vi "max and min of domain and freq.vi"() -> ()   [LabVIEW 2017]
uses:
  <vilib>/measure/maspectr.llb/FFT Power Spectrum and PSD for 1 Chan.vi
  <vilib>/measure/NI_MAPro.lvlib
panel:
  out "min value freq":dbl
  out "max value freq":dbl
  out "main signal":waveform(dbl)[](graph)
  out "power spectrum":cluster{"f0":dbl, "df":dbl, "magnitude":dbl[]}(graph)
  out "min value domain":dbl
  out "max value domain":dbl
  in  "path 4":path
  in  "path 3":path
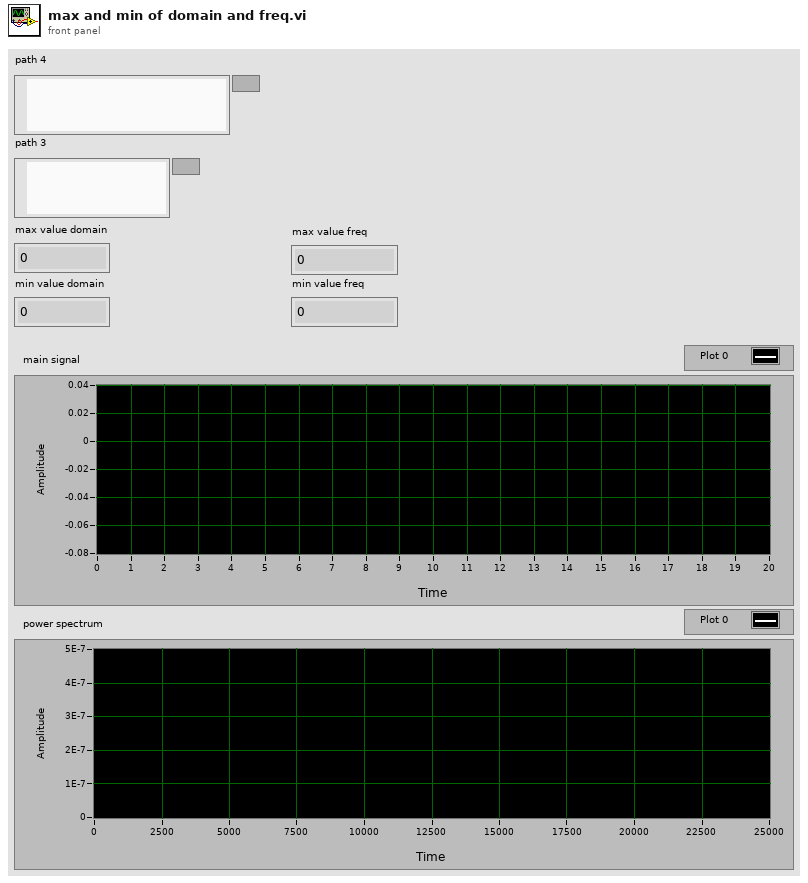
[diagram p1: front panel]
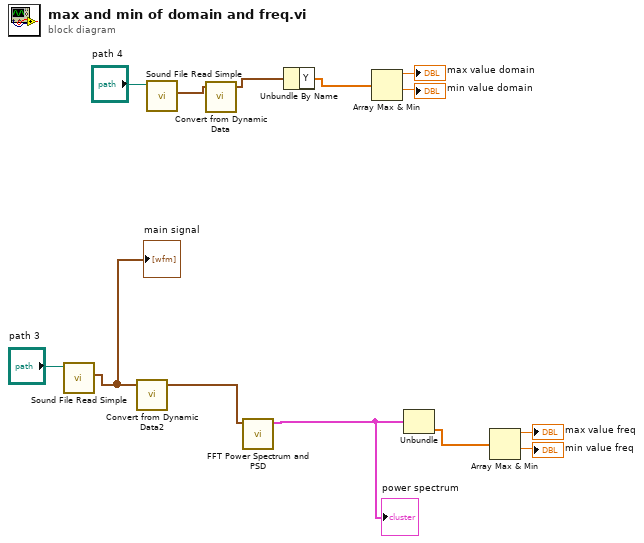
[diagram p0: block diagram]
diagram:
  n1 = call <vilib>:"Sound File Read Simple.vi"("path"="path 3") -> ("data"=w4:waveform(dbl)[])  [unwired: 7 in, 3 out]
  "main signal" <- w4
  n2 = call "Convert from Dynamic Data2"("Dynamic Data Type"=w4) -> ("Waveform"=w6:waveform(dbl))  [unwired: 3 in]
  n3 = call <vilib>:"Sound File Read Simple.vi"("path"="path 4") -> ("data"=w11:waveform(dbl)[])  [unwired: 7 in, 3 out]
  n4 = call "Convert from Dynamic Data"("Dynamic Data Type"=w11) -> ("Waveform"=w10:waveform(dbl))  [unwired: 3 in]
  n5 = call-poly <vilib>:"FFT Power Spectrum and PSD.vi"("time signal"=w6) -> ("Power Spectrum / PSD"=w5:cluster{"f0":dbl, "df":dbl, "magnitude":dbl[]})  [unwired: 7 in, 3 out]
  "power spectrum" <- w5
  n6 = Unbundle By Name(w10) -> ("Y"=w9:dbl[])
  n7 = Array Max & Min(array=w9) -> (max value=→"max value domain":dbl, min value=→"min value domain":dbl)  [unwired: 2 out]
  n8 = Unbundle(w5) -> ("magnitude"=w3:dbl[])  [unwired: 2 out]
  n9 = Array Max & Min(array=w3) -> (max value=→"max value freq":dbl, min value=→"min value freq":dbl)  [unwired: 2 out]
